vi "write_data.vi"(8 "error in (no error)":errorcluster, 10 "data":T1, 11 "PassiveAggressiveRegressor in":refnum<class "PassiveAggressiveRegressor.lvclass">) -> (0 "error out":errorcluster, 3 "PassiveAggressiveRegressor out":refnum<class "PassiveAggressiveRegressor.lvclass">)   [LabVIEW 2020, in "PassiveAggressiveRegressor.lvclass"]
uses:
  PassiveAggressiveRegressor.lvclass
  Controls/passive_agressive_regressor_data.ctl
  PassiveAggressiveRegressor.lvclass/PassiveAggressiveRegressor.ctl
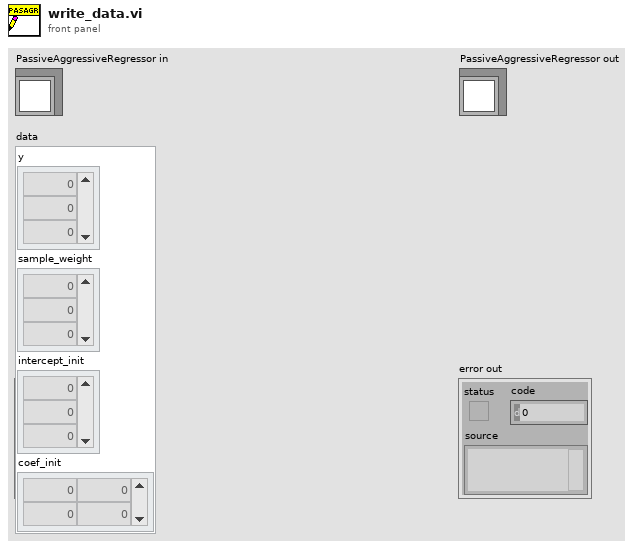
[diagram p1: front panel]
types:
  T1 = typedef "passive_agressive_regressor_data.ctl" = cluster{"y":dbl[], "sample_weight":dbl[], "intercept_init":dbl[], "coef_init":dbl[][]}
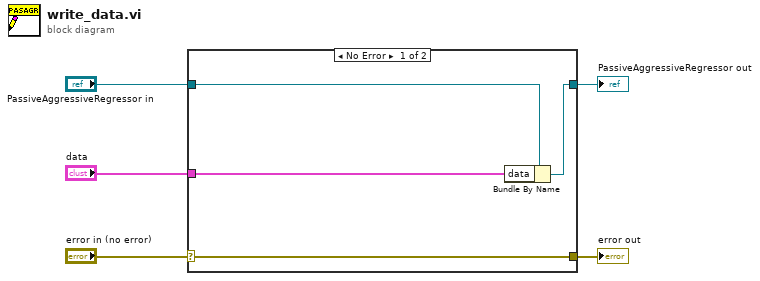
[diagram p0: block diagram]
diagram:
  n1 = case shown="No Error" "error in (no error)" {
    selector: "error in (no error)" -> [w9 w10]
    tunnel: [w9 w10] -> w4
    tunnel: [w7 w11] -> w2
    tunnel: "PassiveAggressiveRegressor in" -> [w8 w11]
    tunnel: "data" -> [w6 _]
    frame No Error {
      n2 = Bundle By Name(cluster=w8, "data"=w6) -> (w7:refnum<class "PassiveAggressiveRegressor.lvclass">)
    }
    frame Error {
    }
  }
  "error out" <- w4
  "PassiveAggressiveRegressor out" <- w2
